vi "Execution Engine.vi"(11 "System":refnum<class "bt_System.lvclass">) -> (0 "error out":errorcluster)   [LabVIEW 2021, in "BT.lvlib" / "bt_System.lvclass"]
uses:
  bt_System.lvclass
  bt_System.lvclass/bt_System.ctl
  Support/Nodes/abs_Node/bt_Node.lvclass
  Support/Nodes/abs_Node/Status.ctl
panel:
  out "Status":T1
  in  "stop":bool
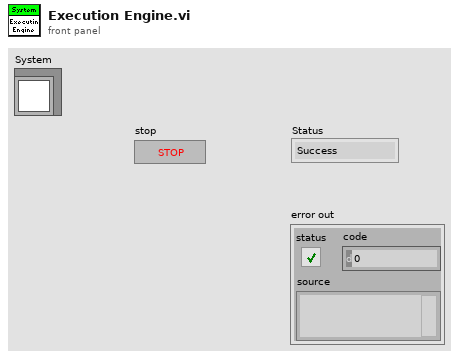
[diagram p1: front panel]
types:
  T1 = typedef "BT.lvlib/bt_Node.lvclass/Status.ctl" = enum16{"Success", "Failure", "Running"}
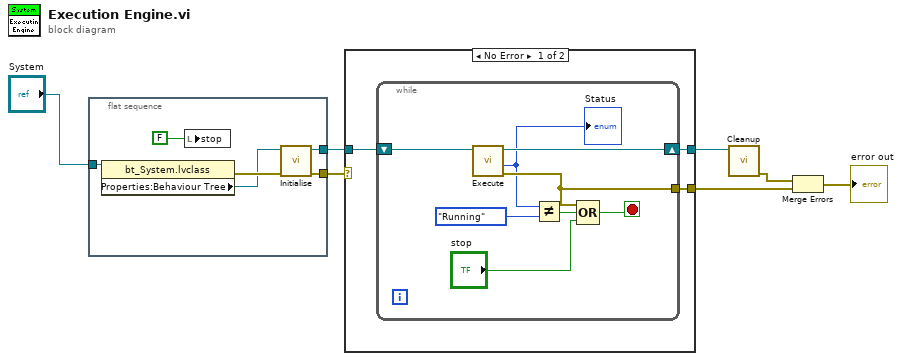
[diagram p0: block diagram]
diagram:
  n1 = flat-sequence {
    tunnel: [w13] -> w7
    tunnel: "System" -> [w11]
    tunnel: [w9] -> w1
    frame #0 {
      n2 = property class="bt_System.lvclass"(reference=w11) -> (error out=w12:errorcluster, "Properties:Behaviour Tree"=w10:refnum<class "bt_Node.lvclass">)  [unwired: 1 in, 1 out]
      n3 = local write "stop"(FALSE ("stop")) -> ()
      n4 = call-dynamic "Initialise.vi"("error in (no error)"=w12, "Node in"=w10) -> ("error out"=w9:errorcluster, "Node out"=w13:refnum<class "bt_Node.lvclass">)  [unwired: 8 in]
    }
  }
  n5 = case shown="No Error" w1 {
    selector: w1 -> [_ w25]
    tunnel: w7 -> [w16 w26]
    tunnel: [w15 w26] -> w6
    tunnel: [w14 w25] -> w3
    frame No Error {
      n6 = while {
        shift-right: [w23] -> w15
        shift-left: w16 -> [w24]
        tunnel: [w18] -> w14
        stop <- w20 stop-if-true
        n7 = call-dynamic "Execute.vi"("Node in"=w24) -> ("error out"=w18:errorcluster, "Status"=w17:T1, "Node out"=w23:refnum<class "bt_Node.lvclass">)  [unwired: 8 in]
        "Status" <- w17
        n8 = Not Equal?(x=w17, y=Status."Running") -> (x != y?=w21:bool)
        n9 = Compound Arithmetic op=OR(w18, w21, "stop") -> (w20:bool)
      }
    }
    frame Error {
    }
  }
  n10 = call-dynamic "Cleanup.vi"("Node in"=w6) -> ("error out"=w4:errorcluster)  [unwired: 9 in, 1 out]
  n11 = Merge Errors(w4, w3) -> (→"error out":errorcluster)
